vi "Single Cam append frame.vi"() -> ()   [LabVIEW 2021]
uses:
  <vilib>/userDefined/High Color/IMAQdx.ctl
  <vilib>/vision/driver/NI_Vision_Acquisition_Software.lvlib
panel:
  in  "Frame rate":dbl
  out "Frames":i32
  out "Image":T1(plugin-control)
  in  "stop":bool
  in  "Image Type":T2 items=["Grayscale (U8)", "Grayscale (I16)", "Grayscale (SGL)", "Complex (CSG)", "RGB (U32)", "HSL (U32)", "RGB (U64)", "Grayscale (U16)"]
  in  "Image Name":string="untitled"
  in  "Session In":T3
  out "Camera Information Array":T4(array[cluster]) {"BusType" format="%x"; "SerialNumberLow" format="%.0x"; "SerialNumberHigh" format="%.0x"}
  in  "Connected Only? (Yes)":bool=TRUE
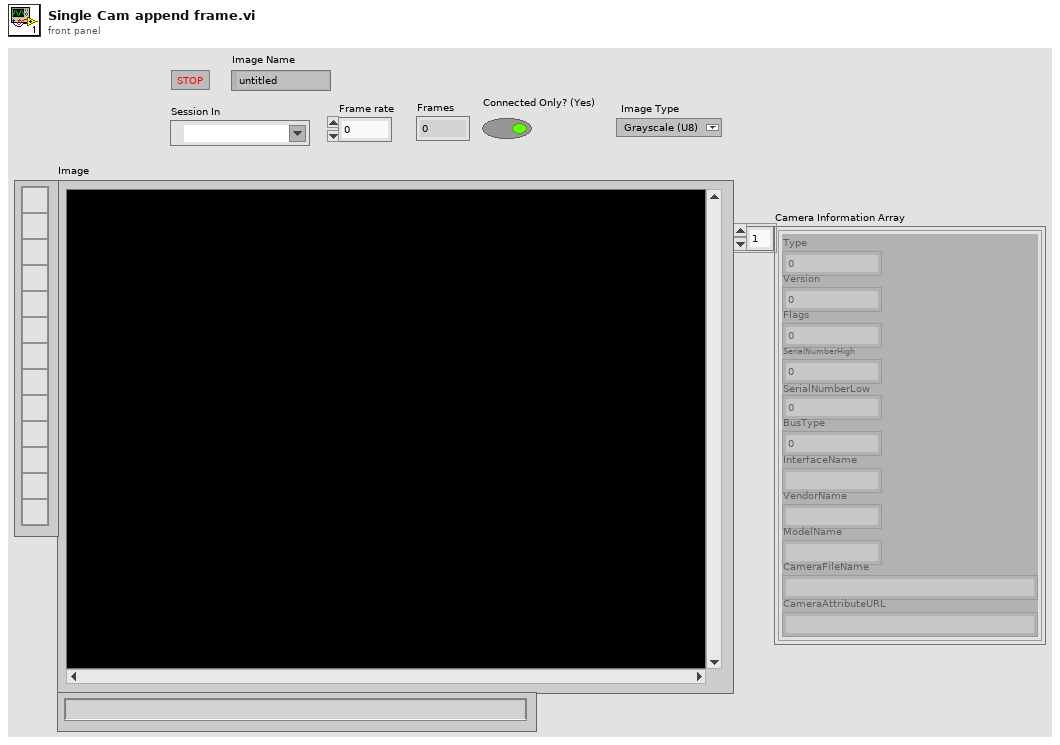
[diagram p1: front panel]
types:
  T1 = typedef "IMAQ Image.ctl" = refnum<image>
  T2 = typedef "Image Type" = u32
  T3 = typedef "IMAQdx.ctl" = refnum<k21>
  T4 = cluster{"Type":u32, "Version":u32, "Flags":u32, "SerialNumberHigh":u32, "SerialNumberLow":u32, "BusType":u32, "InterfaceName":string, "VendorName":string, "ModelName":string, "CameraFileName":string, "CameraAttributeURL":string}[]
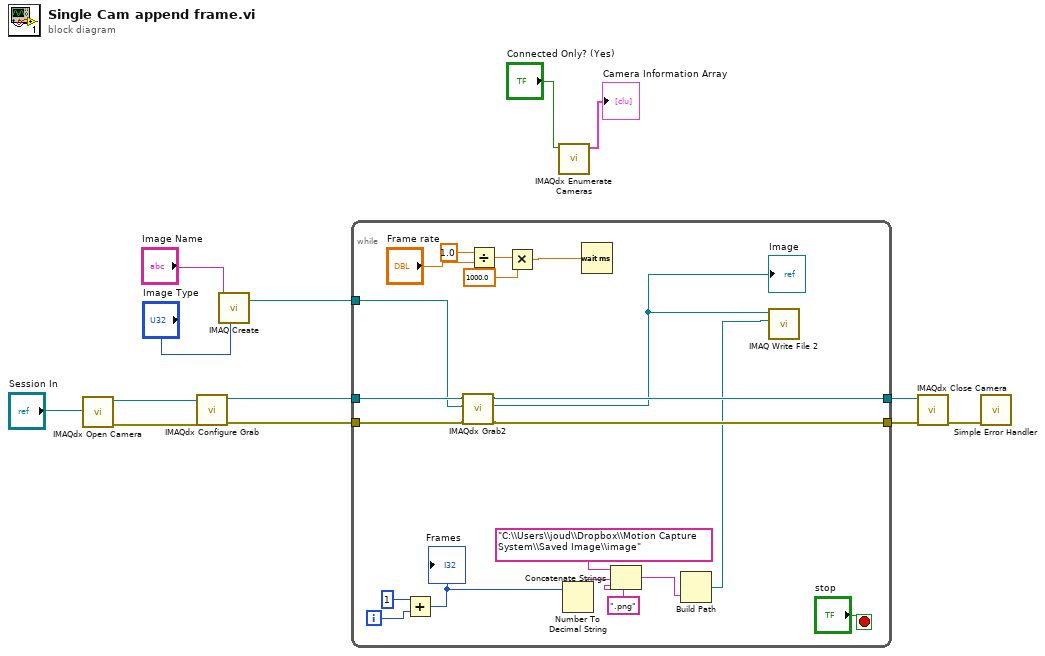
[diagram p0: block diagram]
diagram:
  n1 = call <vilib>:"IMAQdx Open Camera.vi"("Session In"="Session In") -> ("error out"=w9:errorcluster, "Session Out"=w10:T3)  [unwired: 9 in]
  n2 = call <vilib>:"IMAQdx Configure Grab.vi"("error in"=w9, "Session In"=w10) -> ("error out"=w3:errorcluster, "Session Out"=w5:T3)  [unwired: 8 in]
  n3 = call "IMAQ Create"("Image Name"="Image Name", "Image Type"="Image Type") -> ("New Image"=w6:T1)  [unwired: 3 in, 1 out]
  n4 = while {
    tunnel: w6 -> [w30]
    tunnel: w5 -> [w32]
    tunnel: [w28] -> w4
    tunnel: w3 -> [w31]
    tunnel: [w29] -> w1
    i -> [w21]
    stop <- "stop" stop-if-true
    n5 = Add(x=1, y=w21) -> (x+y=w19:i32)
    "Frames" <- w19
    n6 = call <vilib>:"IMAQdx Grab2.vi"("error in"=w31, "Image In"=w30, "Session In"=w32) -> ("error out"=w28:errorcluster, "Image Out"=w27:T1, "Session Out"=w29:T3)  [unwired: 5 in, 1 out]
    "Image" <- w27
    n7 = Divide(x=1.0, y="Frame rate") -> (x/y=w15:dbl)
    n8 = Multiply(x=w15, y=1000.0) -> (x*y=w16:dbl)
    n9 = Number To Decimal String(number=w19) -> (decimal integer string=w26:string)  [unwired: 1 in]
    n10 = Wait (ms)(milliseconds to wait=w16) -> ()  [unwired: 1 out]
    n11 = Concatenate Strings("C:\\Users\\joud\\Dropbox\\Motion Capture System\\Saved Image\\image" ("string"), w26, ".png" ("string")) -> (w23:string)
    n12 = Build Path(name or relative path=w23) -> (appended path=w22:path)  [unwired: 1 in]
    n13 = call-poly "IMAQ Write File 2"("File Path"=w22, "Image"=w27) -> ()  [unwired: 8 in, 2 out]
  }
  n14 = call <vilib>:"IMAQdx Enumerate Cameras.vi"("Connected Only? (Yes)"="Connected Only? (Yes)") -> ("Camera Information Array"=→"Camera Information Array":T4)  [unwired: 9 in, 1 out]
  n15 = call <vilib>:"IMAQdx Close Camera.vi"("error in"=w4, "Session In"=w1) -> ("error out"=w2:errorcluster)  [unwired: 9 in]
  n16 = call <vilib>:"Simple Error Handler.vi"("error in (no error)"=w2) -> ()  [unwired: 4 in, 5 out]
